vi "TimeStampWithMilliseconds.vi"() -> (1 "LabVIEW TimeStamp":timestamp, 3 "Date Formatted with Milliseconds":string)   [LabVIEW 2015]
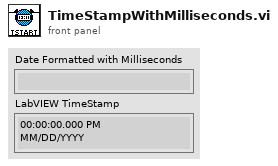
[diagram p1: front panel]
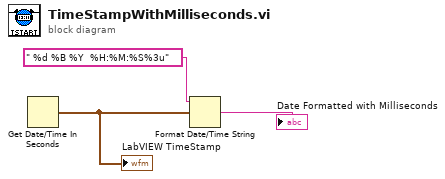
[diagram p0: block diagram]
diagram:
  n1 = Get Date/Time In Seconds() -> (seconds since 1Jan1904=w2:timestamp)
  "LabVIEW TimeStamp" <- w2
  n2 = Format Date/Time String(time format string (%c)=" %d %B %Y  %H:%M:%S%3u", seconds (now)=w2) -> (date/time string=→"Date Formatted with Milliseconds":string)  [unwired: 1 in]
